vi "ConnectedStatusToSLServer.vi"() -> ()   [LabVIEW 2020]
uses:
  <vilib>/Skyline/Tag/Shared/typedefs/DataType.ctl
  StateStartTimeUpdate.ctl
  <vilib>/Skyline/Configuration/Configuration HTTP_class/NI Skyline Configuration HTTP.lvclass/NI Skyline Configuration HTTP.ctl
  <vilib>/Skyline/Configuration/Configuration HTTP_class/Open Configuration HTTP.vi
  <vilib>/Skyline/Configuration/HTTP/Open Configuration (Desktop).vi
  <vilib>/Skyline/Message/HTTP Wrapper/Open (HTTP).vi
  <vilib>/Skyline/Tag/Wrapper/Wrapper HTTP_class/Open Tag HTTP.vi
  <vilib>/Skyline/Tag/Wrapper/Wrapper_class/Write Tag (Timestamp).vi
  <vilib>/nisyscfg/Close (System).vi
  <vilib>/Skyline/Tag/Wrapper/Wrapper_class/Delete Tag (Single).vi
  <vilib>/Skyline/Tag/Wrapper/Wrapper_class/Write Tag (Boolean).vi
  <vilib>/Skyline/Configuration/Configuration HTTP_class/NI Skyline Configuration HTTP.lvclass
  <vilib>/Skyline/Message/HTTP Wrapper/NI Skyline Message HTTP.lvclass
  <vilib>/Skyline/Configuration/Configuration_class/NI Skyline Configuration.lvclass
  <vilib>/Skyline/Tag/Wrapper/Wrapper_class/NI Skyline Tag.lvclass
  <vilib>/Skyline/Tag/Wrapper/Wrapper HTTP_class/NI Skyline Tag HTTP.lvclass
  <vilib>/Skyline/Tag/Shared/NI Skyline Tag.lvlib
  <resource>/objmgr/nisysapi.rc
  <vilib>/nisyscfg/nisyscfg.lvlib
  <vilib>/Skyline/Utilities/NI Skyline Utilities.lvlib
  <vilib>/Skyline/Message/NI Skyline Message.lvclass
panel:
  in  "stop":bool
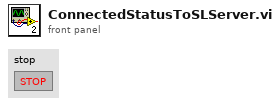
[diagram p1: front panel]
types:
  T1 = typedef "StateStartTimeUpdate.ctl" = enum16{"Init", "UpdateStartTime", "CleanUp"}
  T2 = typedef "NI Skyline Tag.lvlib/DataType.ctl" = enum32{"Double", "I32", "String", "Boolean", "U64", "Timestamp"}
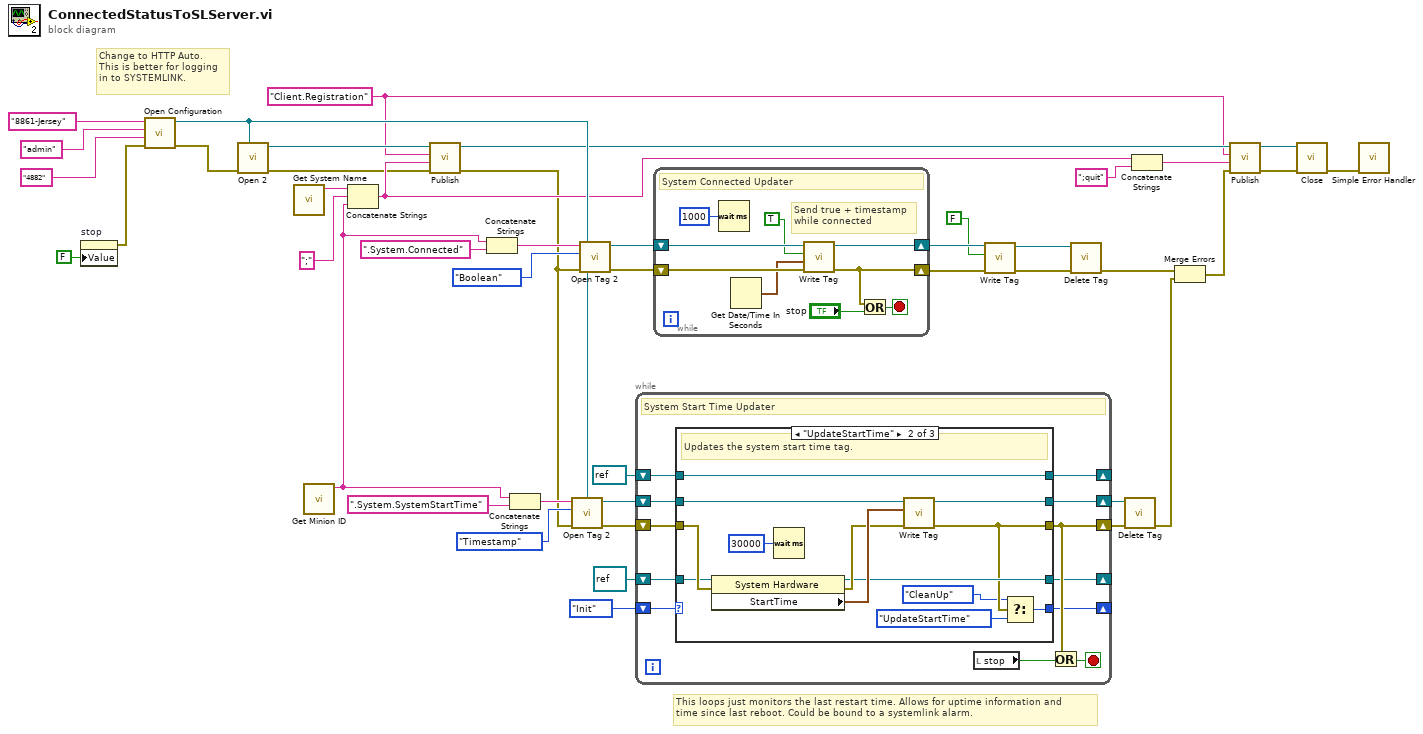
[diagram p0: block diagram]
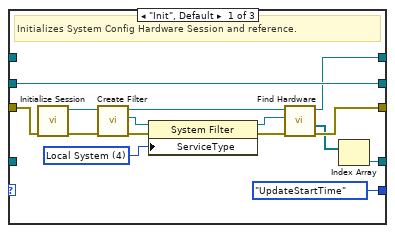
[diagram p2: hidden frame]
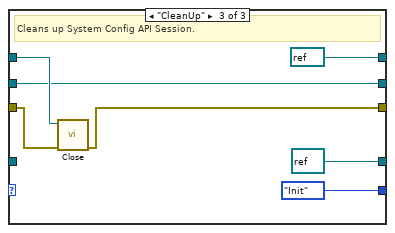
[diagram p3: hidden frame]
diagram:
  w8 = "Client.Registration" ("topic")
  # "Change to HTTP Auto.\nThis is better for logging\nin to SYSTEMLINK."
  # "This loops just monitors the last restart time. Allows for uptime information and\ntime since last reboot. Could be bound to a systemlink alarm."
  n1 = property on="stop" class="Bool (strict)"("Value"=FALSE ("stop")) -> (error out=w18:errorcluster)  [unwired: 2 in, 1 out]
  n2 = call-poly <vilib>:"Open Configuration.vi"("error in (no error)"=w18, "password"="4882", "username"="admin", "server url"="8861-Jersey") -> ("error out"=w19:errorcluster, "configuration"=w20:refnum<class "NI Skyline Configuration HTTP.lvclass">)  [unwired: 6 in]
  n3 = call-poly <vilib>:"Open 2.vi"("configuration"=w20, "error in (no error)"=w19) -> ("error out"=w2:errorcluster, "message session"=w17:refnum<class "NI Skyline Message HTTP.lvclass">)  [unwired: 8 in]
  n4 = call <vilib>:"Get System Name.vi"() -> ("system name"=w16:string)  [unwired: 11 in]
  n5 = call <vilib>:"Get Minion ID.vi"() -> ("minion id"=w15:string)  [unwired: 11 in]
  n6 = Concatenate Strings(w16, ";", w15) -> (w6:string)
  n7 = call-dynamic "Publish.vi"("error in (no error)"=w2, "message"=w6, "topic"=w8, "message session in"=w17) -> ("error out"=w1:errorcluster, "message session out"=w11:refnum<class "NI Skyline Message HTTP.lvclass">)  [unwired: 6 in]
  n8 = Concatenate Strings(w15, ".System.Connected" ("path")) -> (w21:string)
  n9 = Concatenate Strings(w15, ".System.SystemStartTime" ("path")) -> (w22:string)
  n10 = call-poly <vilib>:"Open Tag 2.vi"("configuration"=w20, "error in (no error)"=w1, "Data Type"=DataType."Timestamp", "path"=w22) -> ("error out"=w31:errorcluster, "tag"=w32:refnum<class "NI Skyline Tag.lvclass">)  [unwired: 6 in]
  n11 = call-poly <vilib>:"Open Tag 2.vi"("configuration"=w20, "error in (no error)"=w1, "Data Type"=DataType."Boolean", "path"=w21) -> ("error out"=w39:errorcluster, "tag"=w25:refnum<class "NI Skyline Tag.lvclass">)  [unwired: 6 in]
  n12 = while {
    shift-right: [w55] -> w30
    shift-left: w32 -> [w56]
    shift-right: [w54] -> w29
    shift-left: w31 -> [w53]
    shift-right: [w51] -> _
    shift-left: refnum<k20> refnum ("resource out") -> [w49]
    shift-right: [w50] -> _
    shift-left: StateStartTimeUpdate."Init" -> [w52]
    shift-right: [w48] -> _
    shift-left: refnum<k21> refnum ("Session out") -> [w47]
    stop <- w46 stop-if-true
    # "System Start Time Updater"
    n13 = case shown="\"UpdateStartTime\"" w52 {
      tunnel: w56 -> [w71 w84 w88]
      tunnel: [w71 w83 w88] -> w55
      tunnel: [w61 w75 w86] -> w54
      tunnel: w53 -> [w70 w81 w90]
      tunnel: [w59 w78 refnum<k20> refnum ("resource out")] -> w51
      tunnel: [StateStartTimeUpdate."UpdateStartTime" w73 StateStartTimeUpdate."Init"] -> w50
      tunnel: w49 -> [_ w79 _]
      tunnel: [w57 w76 refnum<k21> refnum ("Session out")] -> w48
      tunnel: w47 -> [_ w76 w91]
      frame "Init", Default {
        w65 = u32 4 items=["NI Network Resource", "NI Real-Time", "NI System Configuration", "NI Web Interface", "Local System", "Local Network Adapter", "Local Time Keeper", "Local Time Reference", "LXI Instrument", "Local FPGA"] ("Service Type")
        # "Initializes System Config Hardware Session and reference."
        n14 = call <vilib>:"Initialize Session.vi"("error in (no error)"=w70) -> ("error out"=w66:errorcluster, "Session out"=w67:refnum<k21>)  [unwired: 9 in]
        n15 = call <vilib>:"Create Filter.vi"("error in (no error)"=w66, "Session in"=w67) -> ("error out"=w68:errorcluster, "Filter out"=w69:refnum<k20>, "Session out"=w62:refnum<k21>)  [unwired: 7 in]
        n16 = property class="System Filter"(reference=w69, error in=w68, "ServiceType"=w65) -> (reference out=w64:refnum<k20>, error out=w63:errorcluster)
        n17 = call <vilib>:"Find Hardware.vi"("error in (no error)"=w63, "Filter in"=w64, "Session in"=w62) -> ("error out"=w61:errorcluster, "Resources out"=w60:refnum<k20>[], "Session out"=w57:refnum<k21>)  [unwired: 5 in, 1 out]
        n18 = Index Array(array=w60) -> (element=w59:refnum<k20>)  [unwired: 1 in]
      }
      frame "UpdateStartTime" {
        # "Updates the system start time tag."
        n19 = property class="System Hardware"(reference=w79, error in=w81) -> (reference out=w78:refnum<k20>, error out=w80:errorcluster, "StartTime"=w82:timestamp)
        n20 = Wait (ms)(milliseconds to wait=u32 30000) -> ()  [unwired: 1 out]
        n21 = call-poly <vilib>:"Write Tag.vi"("error in (no error)"=w80, "value"=w82, "tag in"=w84) -> ("error out"=w75:errorcluster, "tag out"=w83:refnum<class "NI Skyline Tag.lvclass">)  [unwired: 7 in]
        n22 = Select(t=StateStartTimeUpdate."CleanUp", s=w75, f=StateStartTimeUpdate."UpdateStartTime") -> (s? t:f=w73:T1)
      }
      frame "CleanUp" {
        # "Cleans up System Config API Session."
        n23 = call-poly <vilib>:"Close.vi"("error in (no error)"=w90, "Session in"=w91) -> ("error out"=w86:errorcluster)  [unwired: 9 in]
      }
    }
    n24 = local read "stop"() -> (w45:bool)
    n25 = Or(x=w54, y=w45) -> (x .or. y?=w46:bool)
  }
  n26 = while {
    shift-right: [w97] -> w37
    shift-left: w39 -> [w99]
    shift-right: [w98] -> w38
    shift-left: w25 -> [w100]
    stop <- w93 stop-if-true
    # "Send true + timestamp\nwhile connected"
    # "System Connected Updater"
    n27 = Wait (ms)(milliseconds to wait=u32 1000) -> ()  [unwired: 1 out]
    n28 = Get Date/Time In Seconds() -> (seconds since 1Jan1904=w95:timestamp)
    n29 = call-poly <vilib>:"Write Tag.vi"("error in (no error)"=w99, "time stamp"=w95, "value"=TRUE, "tag in"=w100) -> ("error out"=w97:errorcluster, "tag out"=w98:refnum<class "NI Skyline Tag.lvclass">)  [unwired: 6 in]
    n30 = Or(x=w97, y="stop") -> (x .or. y?=w93:bool)
  }
  n31 = call-poly <vilib>:"Write Tag.vi"("error in (no error)"=w37, "value"=FALSE, "tag in"=w38) -> ("error out"=w34:errorcluster, "tag out"=w35:refnum<class "NI Skyline Tag.lvclass">)  [unwired: 7 in]
  n32 = call-poly <vilib>:"Delete Tag.vi"("error in (no error)"=w34, "tag"=w35) -> ("error out"=w13:errorcluster)  [unwired: 9 in]
  n33 = call-poly <vilib>:"Delete Tag.vi"("error in (no error)"=w29, "tag"=w30) -> ("error out"=w12:errorcluster)  [unwired: 9 in]
  n34 = Concatenate Strings(w6, ";quit" ("string")) -> (w5:string)
  n35 = Merge Errors(w13, w12) -> (w9:errorcluster)
  n36 = call-dynamic "Publish.vi"("error in (no error)"=w9, "message"=w5, "topic"=w8, "message session in"=w11) -> ("error out"=w7:errorcluster, "message session out"=w10:refnum<class "NI Skyline Message HTTP.lvclass">)  [unwired: 6 in]
  n37 = call-dynamic <vilib>:"Close.vi"("error in (no error)"=w7, "message session"=w10) -> ("error out"=w3:errorcluster)  [unwired: 9 in]
  n38 = call <vilib>:"Simple Error Handler.vi"("error in (no error)"=w3) -> ()  [unwired: 4 in, 5 out]
